vi "Correct_Losing_Origin_for_Splitting_Problem-1.vi"(4 "error IN":errorcluster, 5 "[IN] # of Correc\nted Longest Track":i32, 6 "[IN] # of Prob\nlem Point Inside":i32, 7 "[IN] Still connected\ntracks in group":T2) -> (0 "error OUT":errorcluster, 1 "[OUT] # of Correc\nted Longest Track":i32, 2 "[OUT] # of Prob\nlem Point Inside":i32, 3 "[OUT] Clusters for Re\nconstructed Tracks":T1)   [LabVIEW 2013]
doc: "Subprogram corrects the following mistake:\ntwo crossing tracks recognised as the single track with the splitting event"
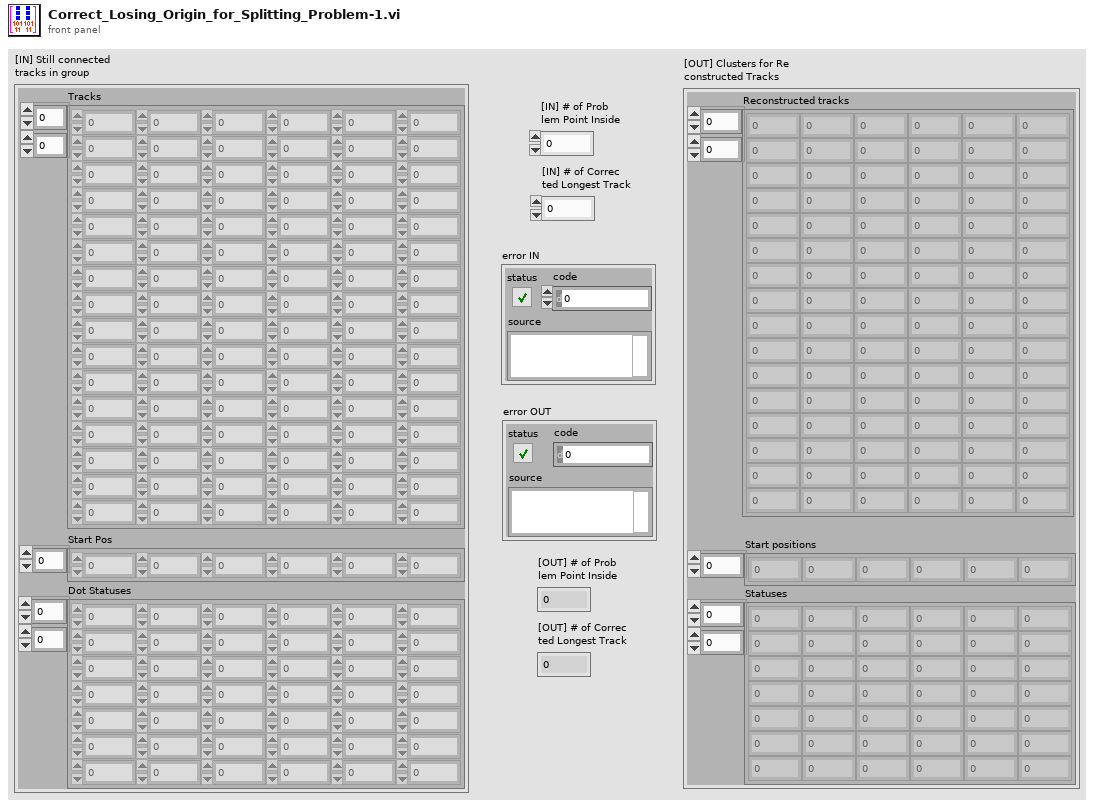
[diagram p1: front panel]
types:
  T1 = cluster{"Reconstructed tracks":dbl[][], "Start positions":i32[], "Statuses":i16[][]}
  T2 = cluster{"Tracks":dbl[][], "Start Pos":i32[], "Dot Statuses":i16[][]}
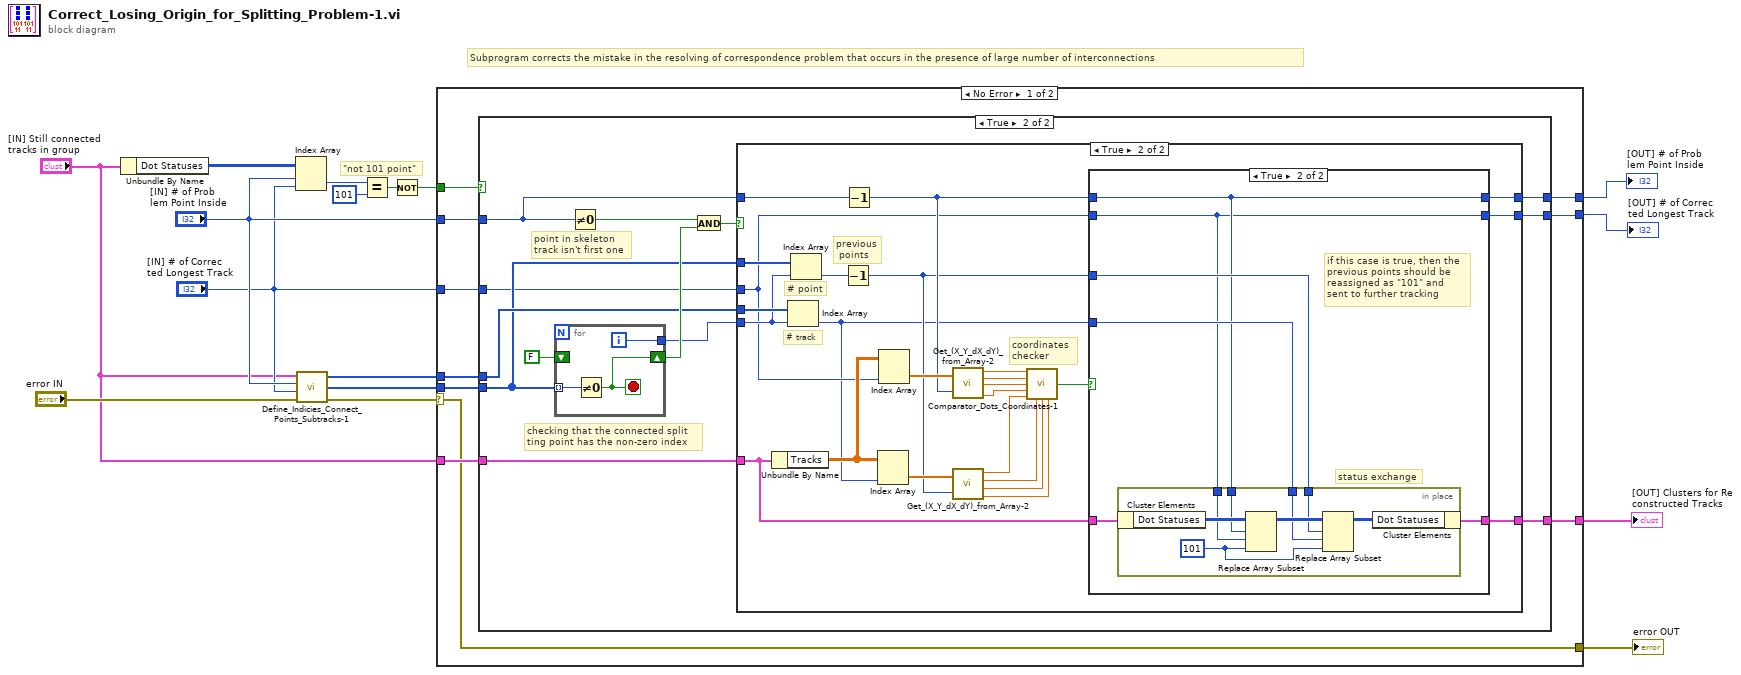
[diagram p0: block diagram]
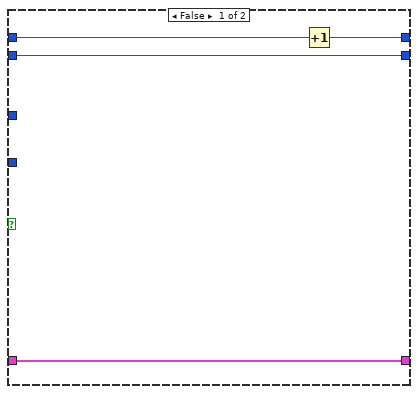
[diagram p4: hidden frame]
diagram:
  # "\"not 101 point\""
  # "Subprogram corrects the mistake in the resolving of correspondence problem that occurs in the presence of large number of interconnections"
  n1 = Unbundle By Name("[IN] Still connected\ntracks in group") -> ("Dot Statuses"=w13:i16[][])
  n2 = Index Array(array=w13, index (row)="[IN] # of Prob\nlem Point Inside", index (col)="[IN] # of Correc\nted Longest Track") -> (element=w16:i16)
  n3 = call "Define_Indicies_Connect_Points_Subtracks-1.vi"("error IN"="error IN", "[IN] Index of track with\n(problem displacement)"="[IN] # of Correc\nted Longest Track", "[IN] Index of problem\ndisplacement inside track"="[IN] # of Prob\nlem Point Inside", "[IN] Track group"="[IN] Still connected\ntracks in group") -> ("error OUT"=w12:errorcluster, "[OUT] Index of \nconnected dots\ninside the track"=w8:i32[], "[OUT] Index of connected\ntracks with problem dot"=w7:i32[])
  n4 = Equal?(x=w16, y=i16 101) -> (x = y?=w11:bool)
  n5 = Not(x=w11) -> (.not. x?=w10:bool)
  n6 = case shown="No Error" w12 {
    selector: w12 -> [w19 w94]
    tunnel: w10 -> [w26 _]
    tunnel: "[IN] # of Prob\nlem Point Inside" -> [w25 w93]
    tunnel: w8 -> [w24 _]
    tunnel: w7 -> [w23 _]
    tunnel: "[IN] # of Correc\nted Longest Track" -> [w22 w92]
    tunnel: "[IN] Still connected\ntracks in group" -> [w21 w95]
    tunnel: [w20 w95] -> w3
    tunnel: [w19 w94] -> w4
    tunnel: [w18 w93] -> w2
    tunnel: [w17 w92] -> w1
    frame No Error {
      n7 = case shown="True" w26 {
        tunnel: w25 -> [w28 w34]
        tunnel: w24 -> [_ w36]
        tunnel: w23 -> [_ w37]
        tunnel: w22 -> [w27 w35]
        tunnel: w21 -> [w29 w33]
        tunnel: [w29 w32] -> w20
        tunnel: [w28 w31] -> w18
        tunnel: [w27 w30] -> w17
        frame False {
        }
        frame True {
          # "point in skeleton \ntrack isn't first one"
          # "checking that the connected split\nting point has the non-zero index"
          n8 = for {
            tunnel: w36 -> [w91] mode=indexing
            shift-right: [w90] -> w41
            shift-left: FALSE -> [_]
            tunnel: [w89] -> w38
            i -> [w89]
            stop <- w90 stop-if-true
            n9 = Not Equal To 0?(x=w91) -> (x != 0?=w90:bool)
          }
          n10 = Not Equal To 0?(x=w34) -> (x != 0?=w40:bool)
          n11 = And(x=w40, y=w41) -> (x .and. y?=w39:bool)
          n12 = case shown="True" w39 {
            tunnel: w38 -> [_ w69]
            tunnel: w37 -> [_ w70]
            tunnel: w36 -> [_ w68]
            tunnel: w35 -> [w43 w52]
            tunnel: w34 -> [w44 w46]
            tunnel: w33 -> [w45 w54]
            tunnel: [w45 w49] -> w32
            tunnel: [w44 w48] -> w31
            tunnel: [w43 w47] -> w30
            frame False {
            }
            frame True {
              # "coordinates \nchecker"
              # "previous\n points"
              # "# point"
              # "# track"
              n13 = Unbundle By Name(w54) -> ("Tracks"=w66:dbl[][])
              n14 = Index Array(array=w70, index=w69) -> (element=w50:i32)
              n15 = Index Array(array=w68, index=w69) -> (element=w67:i32)
              n16 = Decrement(x=w67) -> (x-1=w51:i32)
              n17 = Decrement(x=w46) -> (x-1=w53:i32)
              n18 = Index Array(array=w66, index (col)=w50) -> (element=w64:dbl[])  [unwired: 1 in]
              n19 = Index Array(array=w66, index (col)=w52) -> (element=w65:dbl[])  [unwired: 1 in]
              n20 = call "Get_(X_Y_dX_dY)_from_Array-2.vi"("(X,Y,dX,dY)"=w65, "Index of Displacement"=w53) -> ("X"=w63:dbl, "Y"=w62:dbl, "dX"=w61:dbl, "dY"=w60:dbl)
              n21 = call "Get_(X_Y_dX_dY)_from_Array-2.vi"("(X,Y,dX,dY)"=w64, "Index of Displacement"=w51) -> ("X"=w59:dbl, "Y"=w58:dbl, "dX"=w57:dbl, "dY"=w56:dbl)
              n22 = call "Comparator_Dots_Coordinates-1.vi"("X1"=w63, "Y1"=w62, "(X+dX)1"=w61, "(Y+dY)1"=w60, "X2"=w59, "Y2"=w58, "(X+dX)2"=w57, "(Y+dY)2"=w56) -> ("X1(2)=X2(2),Y1(2)=Y2(2) (2)"=w55:bool)  [unwired: 5 in, 2 out]
              n23 = case shown="True" w55 {
                tunnel: w54 -> [w74 w80]
                tunnel: w53 -> [w73 w76]
                tunnel: w52 -> [w71 w75]
                tunnel: w51 -> [_ w79]
                tunnel: w50 -> [_ w78]
                tunnel: [w74 w77] -> w49
                tunnel: [w72 w76] -> w48
                tunnel: [w71 w75] -> w47
                frame False {
                  n24 = Increment(x=w73) -> (x+1=w72:i32)
                }
                frame True {
                  # "status exchange"
                  # "if this case is true, then the \nprevious points should be \nreassigned as \"101\" and \nsent to further tracking"
                  n25 = in-place {
                    in-place-border: w76 -> [w87]
                    in-place-border: w75 -> [w86]
                    in-place-border: w79 -> [w84]
                    in-place-border: w78 -> [w83]
                    w82 = i16 101 ("new element/subarray")
                    n26 = in-place-cluster #1(w80) -> ("Dot Statuses"=w88:i16[][])
                    n27 = Replace Array Subset(array=w88, new element=w82, index (row)=w87, index (col)=w86) -> (w85:i16[][])
                    n28 = Replace Array Subset(array=w85, new element=w82, index (row)=w84, index (col)=w83) -> (w81:i16[][])
                    n29 = in-place-cluster #1("Dot Statuses"=w81) -> (w77:T2)
                  }
                }
              }
            }
          }
        }
      }
    }
    frame Error {
    }
  }
  "[OUT] Clusters for Re\nconstructed Tracks" <- w3
  "error OUT" <- w4
  "[OUT] # of Prob\nlem Point Inside" <- w2
  "[OUT] # of Correc\nted Longest Track" <- w1
